vi "HandleObservation.vi"(8 "error in (no error)":errorcluster, 11 "S4ACS_GUI in":refnum<class "S4GUI.lvclass">) -> (0 "error out":errorcluster, 3 "S4ACS_GUI out":refnum<class "S4GUI.lvclass">)   [LabVIEW 2018, in "S4GUI.lvclass"]
uses:
  S4GUI.lvclass
  S4GUI.lvclass/S4GUI.ctl
  Server/Server.lvclass/Server.ctl
  Trigger/Trigger.lvclass/Trigger.ctl
  Acquisition/Acquisition.lvclass
  C:/Users/observer/Desktop/Sparc4GUI/SPARC4_GUI/Server/Server.lvclass
  SyncBox/Sync Box.lvclass
  Server/Server.lvclass
  Trigger/Trigger.lvclass
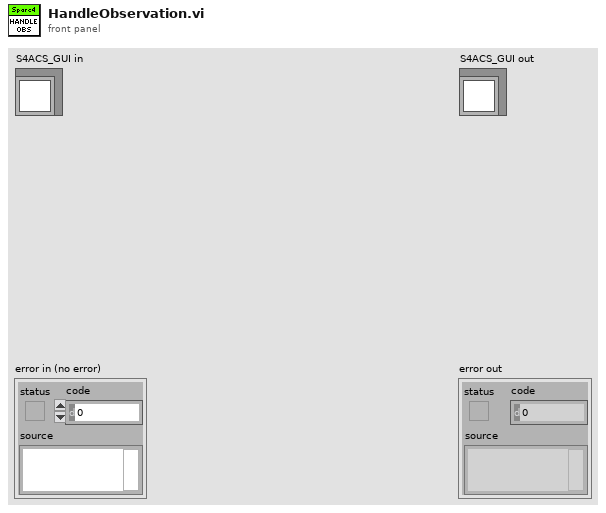
[diagram p1: front panel]
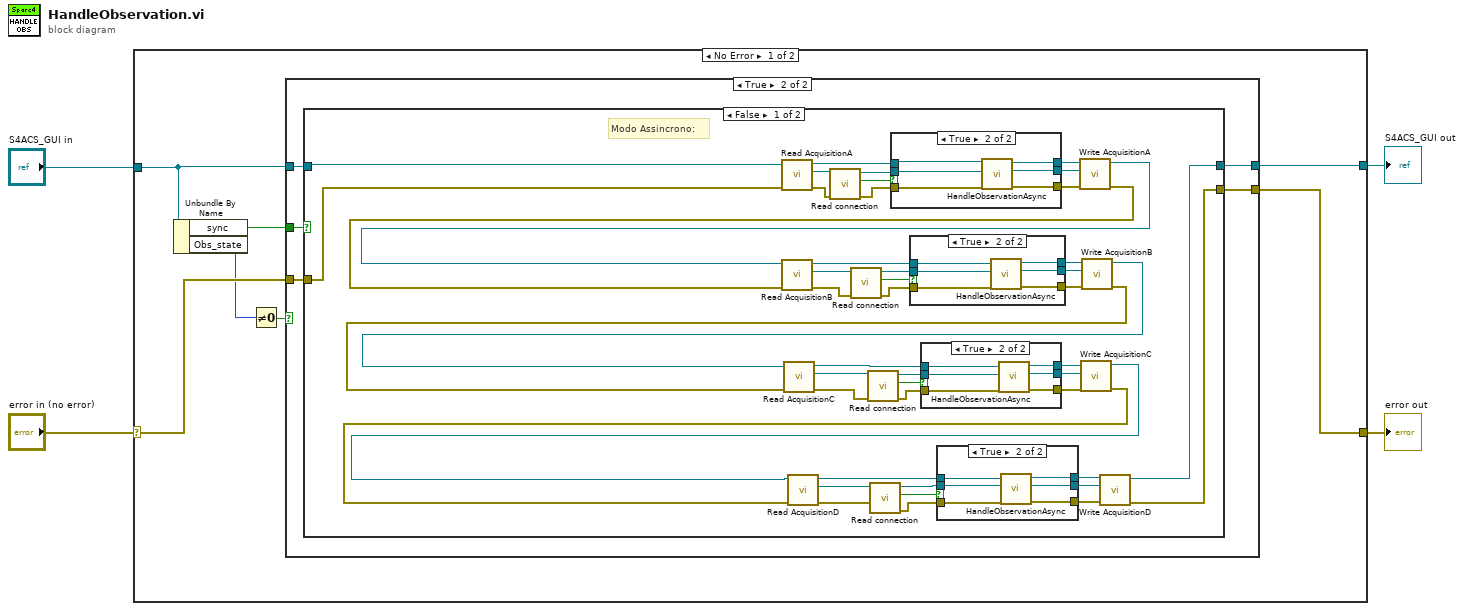
[diagram p0: block diagram]
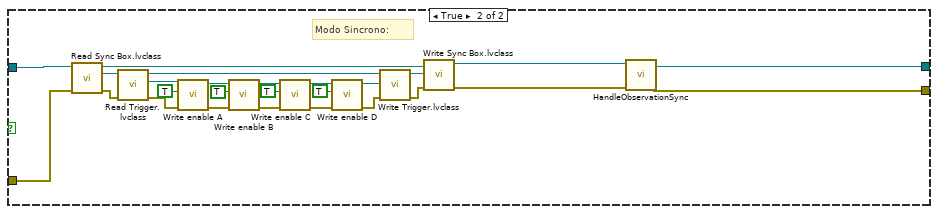
[diagram p7: hidden frame]
diagram:
  n1 = case shown="No Error" "error in (no error)" {
    selector: "error in (no error)" -> [w8 w128]
    tunnel: [w7 w128] -> w3
    tunnel: [w10 w127] -> w1
    tunnel: "S4ACS_GUI in" -> [w11 w127]
    frame No Error {
      n2 = Unbundle By Name(w11) -> ("sync"=w9:bool, "Obs_state"=w6:u32)
      n3 = Not Equal To 0?(x=w6) -> (x != 0?=w5:bool)
      n4 = case shown="True" w5 {
        tunnel: w11 -> [w13 w18]
        tunnel: [w13 w17] -> w10
        tunnel: w9 -> [_ w16]
        tunnel: w8 -> [w12 w15]
        tunnel: [w12 w14] -> w7
        frame False {
        }
        frame True {
          n5 = case shown="False" w16 {
            tunnel: w18 -> [w26 w104]
            tunnel: [w60 w126] -> w17
            tunnel: w15 -> [w25 w103]
            tunnel: [w59 w125] -> w14
            frame False {
              # "Modo Assincrono:"
              n6 = call-dynamic "Read AcquisitionA.vi"("error in (no error)"=w25, "S4ACS_GUI in"=w26) -> ("error out"=w55:errorcluster, "Acquisition.lvclass"=w58:refnum<class "Acquisition.lvclass">, "S4ACS_GUI out"=w64:refnum<class "S4GUI.lvclass">)  [unwired: 7 in]
              n7 = call "Read connection.vi"("error in (no error)"=w55, "Server in"=w58) -> ("error out"=w54:errorcluster, "connection"=w56:bool, "Server out"=w57:refnum<class "Acquisition.lvclass">)  [unwired: 7 in]
              n8 = case shown="True" w56 {
                tunnel: w64 -> [w93 w100]
                tunnel: w57 -> [w94 w99]
                tunnel: w54 -> [w92 w98]
                tunnel: [w93 w97] -> w63
                tunnel: [w94 w96] -> w62
                tunnel: [w92 w95] -> w61
                frame False {
                }
                frame True {
                  n9 = call-dynamic "HandleObservationAsync.vi"("error in (no error)"=w98, "Acquisition.lvclass In"=w99, "S4ACS_GUI in"=w100) -> ("error out"=w95:errorcluster, "Acquisition.lvclass Out"=w96:refnum<class "Acquisition.lvclass">, "S4ACS_GUI out"=w97:refnum<class "S4GUI.lvclass">)  [unwired: 6 in]
                }
              }
              n10 = call-dynamic "Write AcquisitionA.vi"("error in (no error)"=w61, "Acquisition.lvclass"=w62, "S4ACS_GUI in"=w63) -> ("error out"=w23:errorcluster, "S4ACS_GUI out"=w24:refnum<class "S4GUI.lvclass">)  [unwired: 7 in]
              n11 = call "Read AcquisitionB.vi"("error in (no error)"=w23, "S4ACS_GUI in"=w24) -> ("error out"=w49:errorcluster, "Acquisition.lvclass"=w52:refnum<class "Acquisition.lvclass">, "S4ACS_GUI out"=w53:refnum<class "S4GUI.lvclass">)  [unwired: 7 in]
              n12 = call "Read connection.vi"("error in (no error)"=w49, "Server in"=w52) -> ("error out"=w48:errorcluster, "connection"=w50:bool, "Server out"=w51:refnum<class "Acquisition.lvclass">)  [unwired: 7 in]
              n13 = case shown="True" w50 {
                tunnel: w53 -> [w84 w91]
                tunnel: w51 -> [w85 w90]
                tunnel: w48 -> [w83 w89]
                tunnel: [w84 w88] -> w45
                tunnel: [w85 w87] -> w46
                tunnel: [w83 w86] -> w47
                frame False {
                }
                frame True {
                  n14 = call-dynamic "HandleObservationAsync.vi"("error in (no error)"=w89, "Acquisition.lvclass In"=w90, "S4ACS_GUI in"=w91) -> ("error out"=w86:errorcluster, "Acquisition.lvclass Out"=w87:refnum<class "Acquisition.lvclass">, "S4ACS_GUI out"=w88:refnum<class "S4GUI.lvclass">)  [unwired: 6 in]
                }
              }
              n15 = call "Write AcquisitionB.vi"("error in (no error)"=w47, "Acquisition.lvclass"=w46, "S4ACS_GUI in"=w45) -> ("error out"=w21:errorcluster, "S4ACS_GUI out"=w22:refnum<class "S4GUI.lvclass">)  [unwired: 7 in]
              n16 = call-dynamic "Read AcquisitionC.vi"("error in (no error)"=w21, "S4ACS_GUI in"=w22) -> ("error out"=w36:errorcluster, "Acquisition.lvclass"=w37:refnum<class "Acquisition.lvclass">, "S4ACS_GUI out"=w41:refnum<class "S4GUI.lvclass">)  [unwired: 7 in]
              n17 = call "Read connection.vi"("error in (no error)"=w36, "Server in"=w37) -> ("error out"=w42:errorcluster, "connection"=w43:bool, "Server out"=w44:refnum<class "Acquisition.lvclass">)  [unwired: 7 in]
              n18 = case shown="True" w43 {
                tunnel: w41 -> [w75 w82]
                tunnel: w44 -> [w76 w81]
                tunnel: w42 -> [w74 w80]
                tunnel: [w75 w79] -> w40
                tunnel: [w76 w78] -> w39
                tunnel: [w74 w77] -> w38
                frame False {
                }
                frame True {
                  n19 = call-dynamic "HandleObservationAsync.vi"("error in (no error)"=w80, "Acquisition.lvclass In"=w81, "S4ACS_GUI in"=w82) -> ("error out"=w77:errorcluster, "Acquisition.lvclass Out"=w78:refnum<class "Acquisition.lvclass">, "S4ACS_GUI out"=w79:refnum<class "S4GUI.lvclass">)  [unwired: 6 in]
                }
              }
              n20 = call-dynamic "Write AcquisitionC.vi"("error in (no error)"=w38, "Acquisition.lvclass"=w39, "S4ACS_GUI in"=w40) -> ("error out"=w19:errorcluster, "S4ACS_GUI out"=w20:refnum<class "S4GUI.lvclass">)  [unwired: 7 in]
              n21 = call-dynamic "Read AcquisitionD.vi"("error in (no error)"=w19, "S4ACS_GUI in"=w20) -> ("error out"=w31:errorcluster, "Acquisition.lvclass"=w30:refnum<class "Acquisition.lvclass">, "S4ACS_GUI out"=w32:refnum<class "S4GUI.lvclass">)  [unwired: 7 in]
              n22 = call "Read connection.vi"("error in (no error)"=w31, "Server in"=w30) -> ("error out"=w33:errorcluster, "connection"=w34:bool, "Server out"=w35:refnum<class "Acquisition.lvclass">)  [unwired: 7 in]
              n23 = case shown="True" w34 {
                tunnel: w32 -> [w66 w73]
                tunnel: w35 -> [w67 w72]
                tunnel: w33 -> [w65 w71]
                tunnel: [w66 w70] -> w29
                tunnel: [w67 w69] -> w28
                tunnel: [w65 w68] -> w27
                frame False {
                }
                frame True {
                  n24 = call-dynamic "HandleObservationAsync.vi"("error in (no error)"=w71, "Acquisition.lvclass In"=w72, "S4ACS_GUI in"=w73) -> ("error out"=w68:errorcluster, "Acquisition.lvclass Out"=w69:refnum<class "Acquisition.lvclass">, "S4ACS_GUI out"=w70:refnum<class "S4GUI.lvclass">)  [unwired: 6 in]
                }
              }
              n25 = call-dynamic "Write AcquisitionD.vi"("error in (no error)"=w27, "Acquisition.lvclass"=w28, "S4ACS_GUI in"=w29) -> ("error out"=w59:errorcluster, "S4ACS_GUI out"=w60:refnum<class "S4GUI.lvclass">)  [unwired: 7 in]
            }
            frame True {
              # "Modo Sincrono:"
              n26 = call-dynamic "Read Sync Box.lvclass.vi"("error in (no error)"=w103, "SPARC4_AC in"=w104) -> ("error out"=w115:errorcluster, "Sync Box.lvclass"=w124:refnum<class "Sync Box.lvclass">, "SPARC4_AC out"=w116:refnum<class "S4GUI.lvclass">)  [unwired: 7 in]
              n27 = call-dynamic "Read Trigger.lvclass.vi"("error in (no error)"=w115, "Sync Box in"=w124) -> ("error out"=w114:errorcluster, "Trigger.lvclass"=w123:refnum<class "Trigger.lvclass">, "Sync Box out"=w121:refnum<class "Sync Box.lvclass">)  [unwired: 7 in]
              n28 = call "Write enable A.vi"("error in (no error)"=w114, "enable A"=TRUE, "Trigger in"=w123) -> ("error out"=w113:errorcluster, "Trigger out"=w122:refnum<class "Trigger.lvclass">)  [unwired: 7 in]
              n29 = call "Write enable B.vi"("error in (no error)"=w113, "enable B"=TRUE, "Trigger in"=w122) -> ("error out"=w112:errorcluster, "Trigger out"=w120:refnum<class "Trigger.lvclass">)  [unwired: 7 in]
              n30 = call "Write enable C.vi"("error in (no error)"=w112, "enable C"=TRUE, "Trigger in"=w120) -> ("error out"=w111:errorcluster, "Trigger out"=w119:refnum<class "Trigger.lvclass">)  [unwired: 7 in]
              n31 = call "Write enable D.vi"("error in (no error)"=w111, "enable D"=TRUE, "Trigger in"=w119) -> ("error out"=w110:errorcluster, "Trigger out"=w118:refnum<class "Trigger.lvclass">)  [unwired: 7 in]
              n32 = call-dynamic "Write Trigger.lvclass.vi"("error in (no error)"=w110, "Trigger.lvclass"=w118, "Sync Box in"=w121) -> ("error out"=w109:errorcluster, "Sync Box out"=w117:refnum<class "Sync Box.lvclass">)  [unwired: 7 in]
              n33 = call-dynamic "Write Sync Box.lvclass.vi"("error in (no error)"=w109, "Sync Box.lvclass"=w117, "SPARC4_AC in"=w116) -> ("error out"=w102:errorcluster, "SPARC4_AC out"=w101:refnum<class "S4GUI.lvclass">)  [unwired: 7 in]
              n34 = call-dynamic "HandleObservationSync.vi"("error in (no error)"=w102, "S4ACS_GUI in"=w101) -> ("error out"=w125:errorcluster, "S4ACS_GUI out"=w126:refnum<class "S4GUI.lvclass">)  [unwired: 8 in]
            }
          }
        }
      }
    }
    frame Error {
    }
  }
  "error out" <- w3
  "S4ACS_GUI out" <- w1
